vi "worksheet repeat rows.vi"(8 "error in (no error)":errorcluster, 9 "last_row":u32, 10 "first_row":u32, 11 "worksheet":u32) -> (0 "error out":errorcluster, 3 "function return":u32(ring))   [LabVIEW 2015, in "xlsxwriter.lvlib"]
doc: "lxw_error worksheet_repeat_rows(lxw_worksheet worksheet, lxw_row_t first_row, lxw_row_t last_row);"
uses:
  xlsxwriter.lvlib
  xlsxwriter.dll
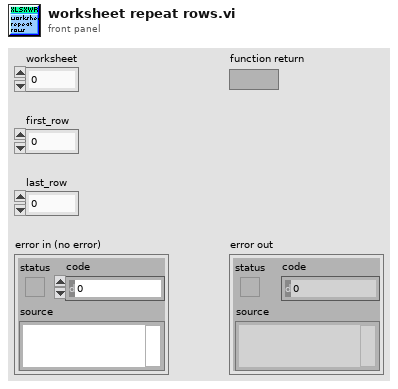
[diagram p1: front panel]
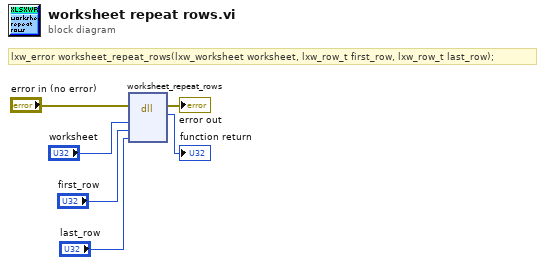
[diagram p0: block diagram]
diagram:
  # "lxw_error worksheet_repeat_rows(lxw_worksheet worksheet, lxw_row_t first_row, lxw_row_t last_row);"
  n1 = dll-call lib="C:/Users/WDAGUtilityAccount/Desktop/lv_vis_added_cell/xlsxwriter.*" fn="worksheet_repeat_rows"(error in="error in (no error)", "worksheet"="worksheet", "first_row"="first_row", "last_row"="last_row") -> (error out=→"error out":errorcluster, →"function return":u32)  [unwired: 5 in, 1 out]
